vi "PH_Connection.Ping Device.vi"(1 "IP":string) -> (0 "successfully pinged?":bool)   [LabVIEW 2014, in "PH_Common.lvlib"]
uses:
  PH_Common.lvlib
panel:
  out "Status (.Net)":i32(ring) items=["Success"=0, "DestinationNetworkUnreachable"=11002, "DestinationHostUnreachable"=11003, "DestinationProhibited, DestinationProtocolUnreachable"=11004, "DestinationPortUnreachable"=11005, "NoResources"=11006, "BadOption"=11007, "HardwareError"=11008, "PacketTooBig"=11009, "TimedOut"=11010, "BadRoute"=11012, "TtlExpired"=11013, "TtlReassemblyTimeExceeded"=11014, "ParameterProblem"=11015, "SourceQuench"=11016, "BadDestination"=11018, "DestinationUnreachable"=11040, "TimeExceeded"=11041, "BadHeader"=11042, "UnrecognizedNextHeader"=11043, "IcmpError"=11044, "DestinationScopeMismatch"=11045, "Unknown"=-1]
  out "error out":errorcluster
  in  "error in (no error)":errorcluster
  out "Output (DOS)":string
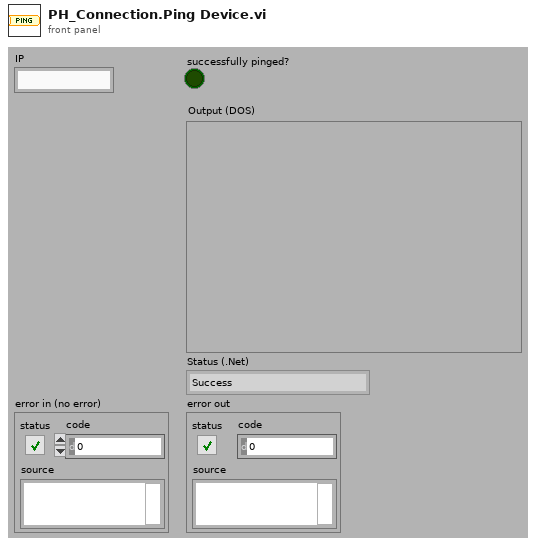
[diagram p1: front panel]
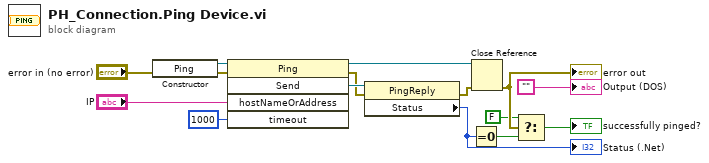
[diagram p0: block diagram]
diagram:
  n1 = constructor class="Ping"(error in="error in (no error)") -> (reference out=w9:refnum<k24>, error out=w8:errorcluster)  [unwired: 2 in, 1 out]
  n2 = invoke class="Ping" method="Send"(reference=w9, error in=w8, "hostNameOrAddress"="IP", "timeout"=1000) -> (reference out=w7:refnum<k24>, error out=w4:errorcluster, "Send"=w5:refnum<k24>)  [unwired: 1 in, 2 out]
  n3 = property class="PingReply"(reference=w5, error in=w4) -> (error out=w3:errorcluster, "Status"=w10:i32)  [unwired: 1 out]
  "Status (.Net)" <- w10
  n4 = Equal To 0?(x=w10) -> (x = 0?=w1:bool)
  n5 = Close Reference(reference=w7, error in (no error)=w3) -> (error out=w11:errorcluster)
  "error out" <- w11
  n6 = Select(t=FALSE, s=w11, f=w1) -> (s? t:f=→"successfully pinged?":bool)
  "Output (DOS)" <- ""
